vi "Stream Length.vi"(8 "error in (no error)":errorcluster, 11 "Streamable Response in":refnum<class "Streamable Response.lvclass">) -> (0 "error out":errorcluster, 2 "Stream Length":i64, 3 "Streamable Response out":refnum<class "Streamable Response.lvclass">)   [LabVIEW 2020, in "HTTP Utils.lvlib" / "Streamable Response.lvclass"]
uses:
  Streamable Response.lvclass
  Streamable Response.lvclass/Streamable Response.ctl
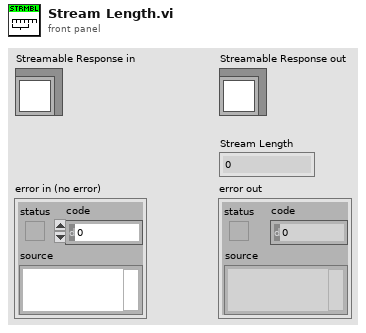
[diagram p1: front panel]
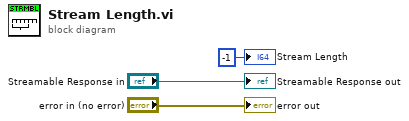
[diagram p0: block diagram]
diagram:
  "error out" <- "error in (no error)"
  "Streamable Response out" <- "Streamable Response in"
  "Stream Length" <- i64 -1 ("Stream Length")
